vi "Main.vi"() -> ()   [LabVIEW 2020, in "Model.lvlib"]
doc: "This template is based off of the Queued Message Handler design pattern and the Queued Message Handler project template that ships with LabVIEW.\n\nThe main difference is that the queue is private to this module and communication between modules is performed via Broadcast and Request events.\n\nRequest events are wrapped in public API methods and are handled in the Event Handling Loop (EHL) of this VI. Any module can register for Broadcast events sent by this module. The EHL generates messages based on user interface actions.\n\nThe Message Handling Loop (MHL) processes messages generated by the EHL, or by other messages. The messages are string values, so new messages can be added easily to the Message Cases case structure in the MHL. Each message cluster can also provide an optional value for Message Data, which is a variant that can be converted to whatever message-specific data is required.\n_____\nBased on Delacor QMH Project Template 4.2.1.64."
uses:
  Model.lvlib
  <vilib>/Delacor/Delacor QMH/Libraries/Module Admin_class/Delacor_lib_QMH_Module Admin.lvclass
  Module Data--cluster.ctl
  <vilib>/Delacor/Delacor QMH/Libraries/Message Queue_class/Delacor_lib_QMH_Message Queue.lvclass/Delacor_lib_QMH_Message Queue.ctl
  Stop Argument--cluster.ctl
  <vilib>/Delacor/Delacor QMH/Libraries/Module Admin_class/Delacor_lib_QMH_Module Admin.lvclass/Delacor_lib_QMH_Module Admin.ctl
  <vilib>/Delacor/Delacor QMH/Libraries/Message Queue_class/Delacor_lib_QMH_Enqueue Message (Single).vi
  <vilib>/Delacor/Delacor QMH/Libraries/Module Admin_class/Delacor_lib_QMH_Get External Launch.vi
  <vilib>/Utility/error.llb/Error Cluster From Error Code.vi
  <vilib>/ErrorRing/Error Ring.xnode
  <vilib>/Delacor/Delacor QMH/Libraries/Message Queue_class/Delacor_lib_QMH_Message Queue.lvclass
  Stock/Stock.lvlib
  Display/Display.lvlib
  Keypad/Keypad.lvlib
  Money/Money.lvlib
panel:
  in  "Power":bool
  in  "Simulate MHL Error":bool
  in  "Simulate EHL Error":bool
  in  "Module Admin":refnum<class "Delacor_lib_QMH_Module Admin.lvclass">
  out "Status":string
  out "error out":errorcluster
  # "https://www.youtube.com/tomslabviewadventure | DQMH Vending Machine"
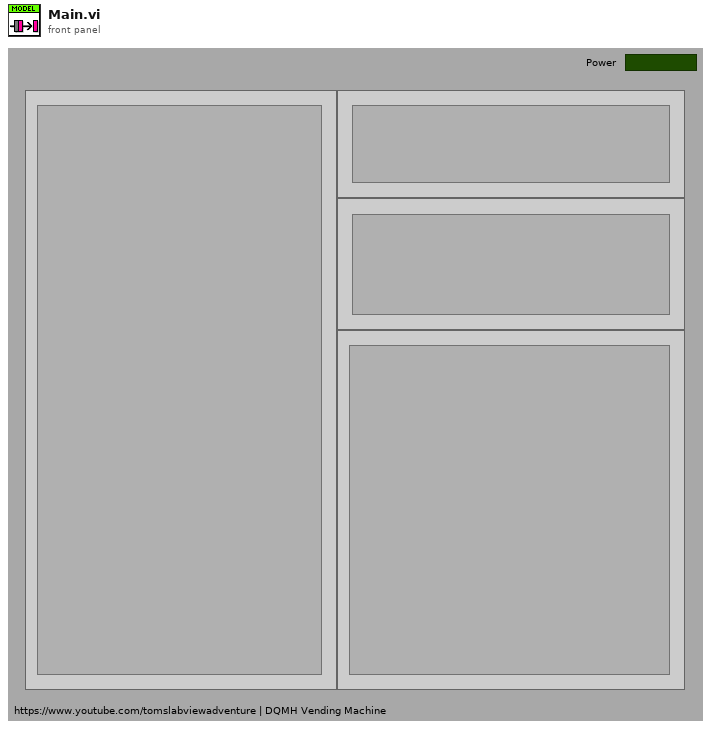
[diagram p1: front panel]
types:
  T1 = typedef "Model.lvlib/Request Events--cluster.ctl" = cluster{"Stop Module":refnum<user-event>, "Show Panel":refnum<user-event>, "Hide Panel":refnum<user-event>, "Get Module Execution Status":refnum<user-event>, "Show Diagram":refnum<user-event>}
  T2 = typedef "Stock.lvlib/Broadcast Events--cluster.ctl" = cluster{"Module Did Init":refnum<user-event>, "Status Updated":refnum<user-event>, "Error Reported":refnum<user-event>, "Module Did Stop":refnum<user-event>, "Update Module Execution Status":refnum<user-event>}
  T3 = typedef "Display.lvlib/Broadcast Events--cluster.ctl" = cluster{"Module Did Init":refnum<user-event>, "Status Updated":refnum<user-event>, "Error Reported":refnum<user-event>, "Module Did Stop":refnum<user-event>, "Update Module Execution Status":refnum<user-event>}
  T4 = typedef "Keypad.lvlib/Broadcast Events--cluster.ctl" = cluster{"Module Did Init":refnum<user-event>, "Status Updated":refnum<user-event>, "Error Reported":refnum<user-event>, "Module Did Stop":refnum<user-event>, "Update Module Execution Status":refnum<user-event>, "Product Selected":refnum<user-event>, "Cancel Request":refnum<user-event>}
  T5 = typedef "Money.lvlib/Broadcast Events--cluster.ctl" = cluster{"Module Did Init":refnum<user-event>, "Status Updated":refnum<user-event>, "Error Reported":refnum<user-event>, "Module Did Stop":refnum<user-event>, "Update Module Execution Status":refnum<user-event>, "Money Entered":refnum<user-event>, "Money Refunded":refnum<user-event>}
  T6 = typedef "Model.lvlib/Module Data--cluster.ctl" = cluster{"Status":string}
  T7 = enum32{"invalid lock state", "Not Locked", "Locked (No Password)", "Password-protected"}
  T8 = typedef "Model.lvlib/Stop Argument--cluster.ctl" = cluster{"Origin":string, "Exit via Stop Module Req?":bool, "Wait for Module to stop?":bool}
  T9 = enum32{"Invalid", "Standard", "Closed", "Hidden", "Minimized", "Maximized"}
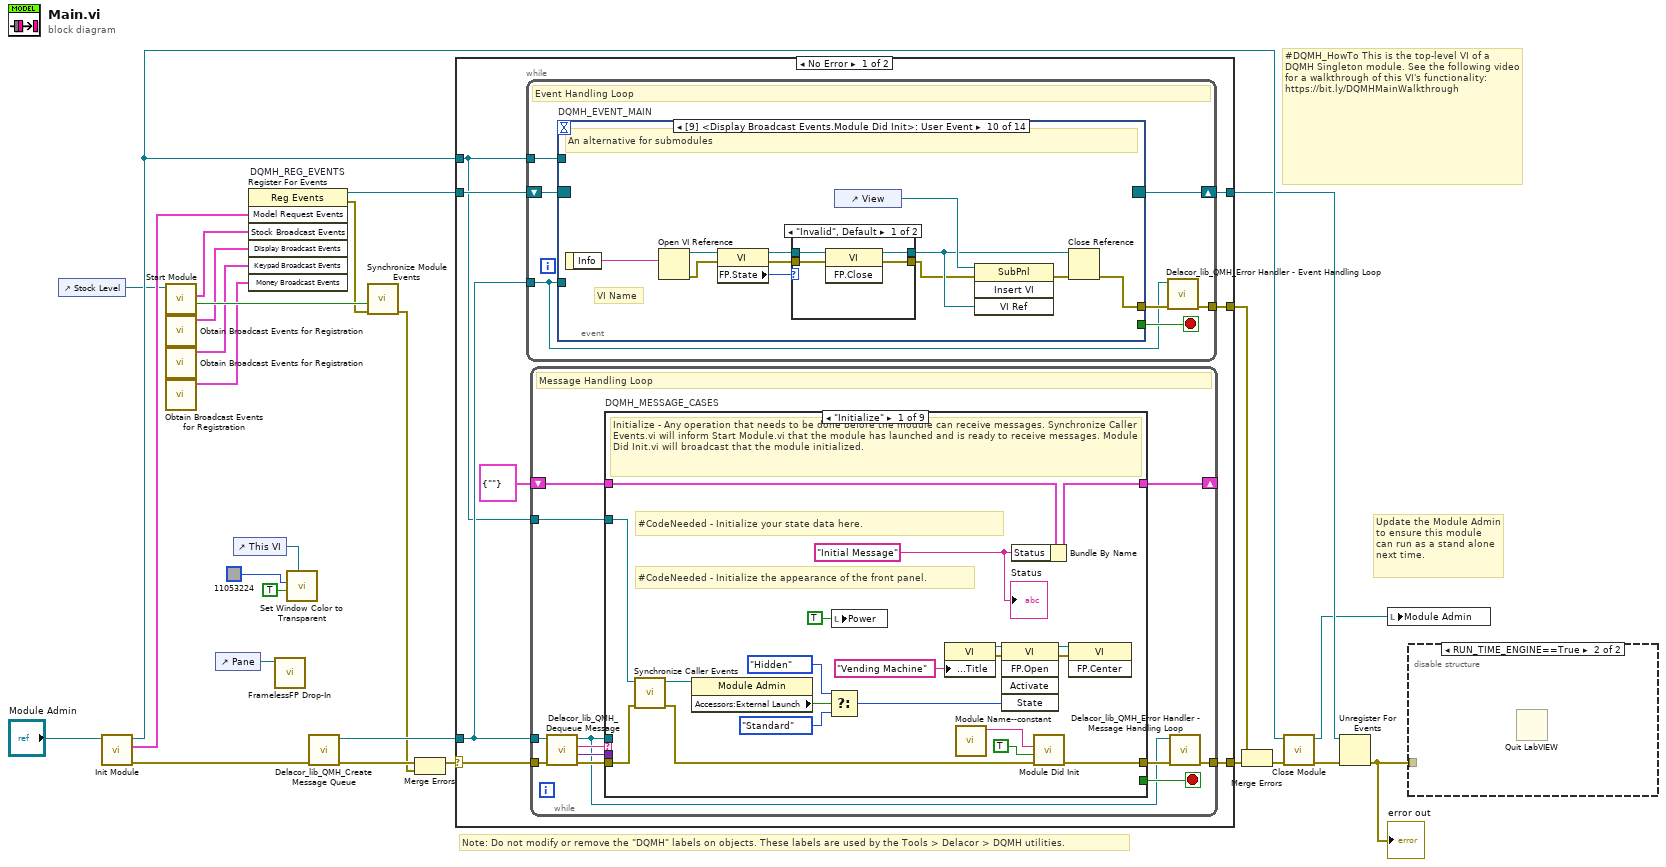
[diagram p0: block diagram]
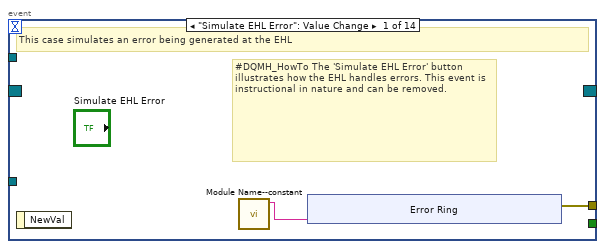
[diagram p3: hidden frame]
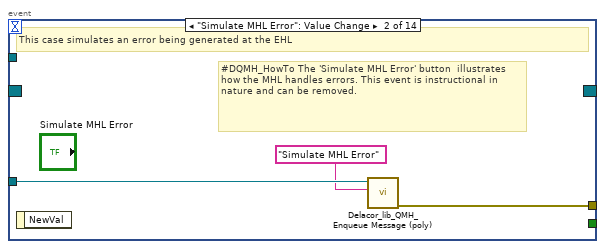
[diagram p4: hidden frame]
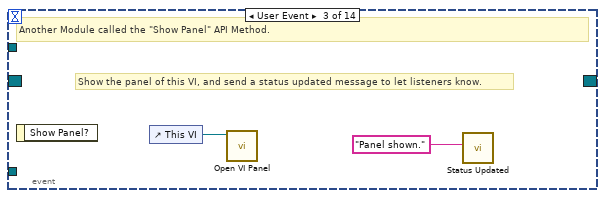
[diagram p5: hidden frame]
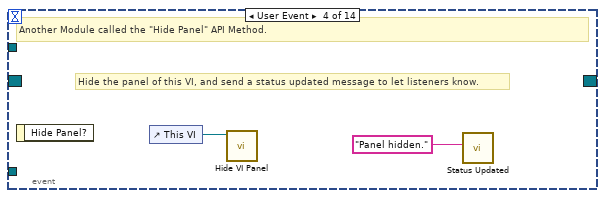
[diagram p6: hidden frame]
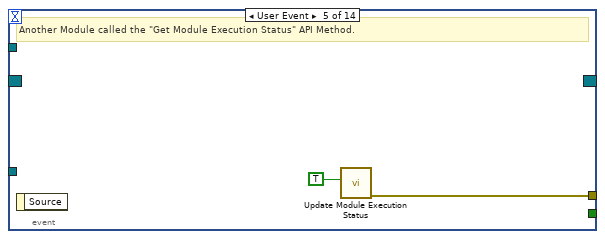
[diagram p7: hidden frame]
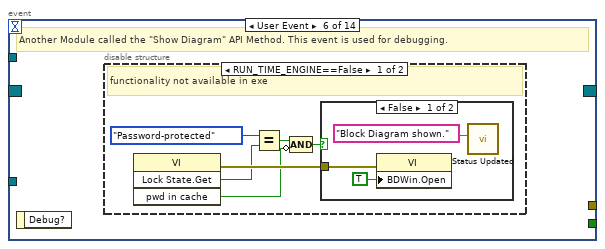
[diagram p8: hidden frame]
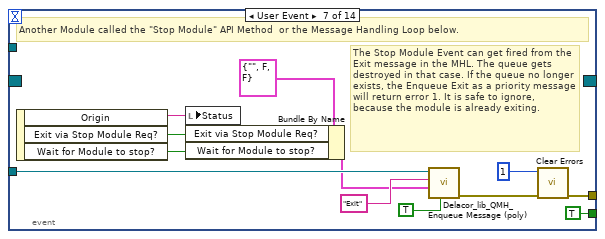
[diagram p11: hidden frame]
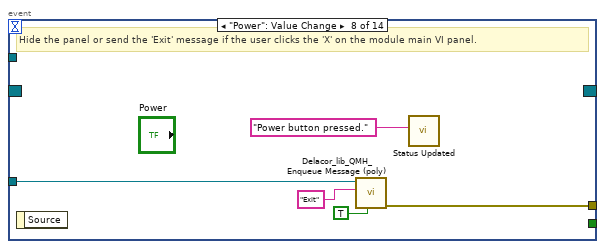
[diagram p12: hidden frame]
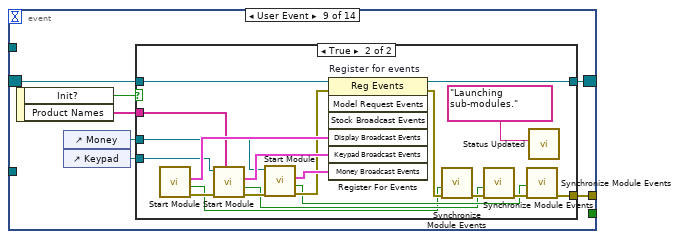
[diagram p13: hidden frame]
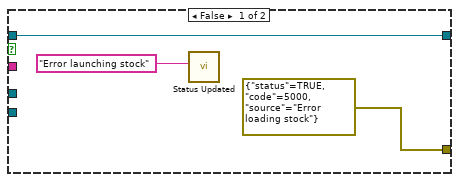
[diagram p14: hidden frame]
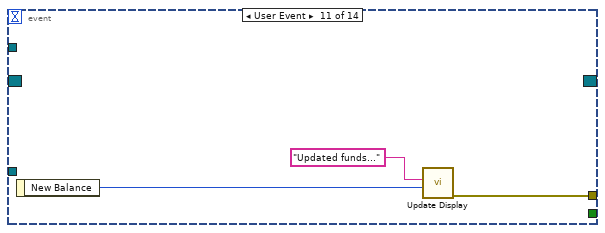
[diagram p16: hidden frame]
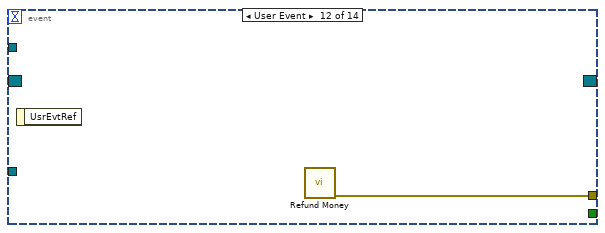
[diagram p17: hidden frame]
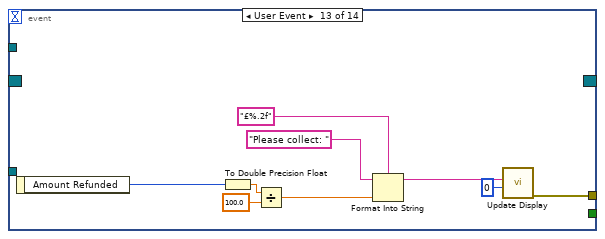
[diagram p18: hidden frame]
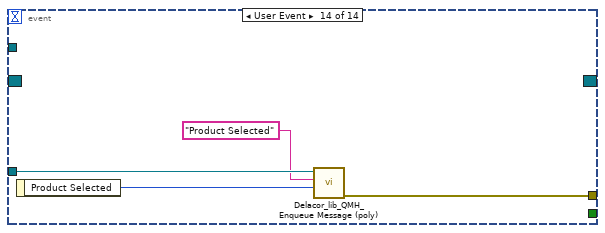
[diagram p19: hidden frame]
diagram:
  # "#DQMH_HowTo This is the top-level VI of a DQMH Singleton module. See the following video for a walkthrough of this VI's functionality: https://bit.ly/DQMHMainWalkthrough"
  # "Note: Do not modify or remove the \"DQMH\" labels on objects. These labels are used by the Tools > Delacor > DQMH utilities."
  # "Update the Module Admin to ensure this module can run as a stand alone next time."
  n1 = control-ref of="Stock Level"() -> (w6:refnum<vi>)
  n2 = call "Init Module.vi"("Singleton Module Admin in"="Module Admin") -> ("error out"=w26:errorcluster, "Model Request Events"=w17:T1, "Singleton Module Admin out"=w20:refnum<class "Delacor_lib_QMH_Module Admin.lvclass">)  [unwired: 8 in]
  n3 = call "Start Module.vi"("Subpanel Ref"=w6) -> ("Wait for Event Sync?"=w12:bool, "Stock Broadcast Events"=w13:T2)  [unwired: 7 in, 2 out]
  n4 = call "Obtain Broadcast Events for Registration.vi"() -> ("Display Broadcast Events"=w9:T3)  [unwired: 9 in, 2 out]
  n5 = call "Obtain Broadcast Events for Registration.vi"() -> ("Keypad Broadcast Events"=w8:T4)  [unwired: 9 in, 2 out]
  n6 = call "Obtain Broadcast Events for Registration.vi"() -> ("Money Broadcast Events"=w7:T5)  [unwired: 9 in, 2 out]
  n7 = control-ref of="Pane"() -> (w4:refnum<vi>)
  n8 = control-ref of="This VI"() -> (w1:refnum<vi>)
  n9 = register-events "DQMH_REG_EVENTS"(w17, w13, w9, w8, w7) -> (reference out=w18:refnum<event-registration>, error out=w11:errorcluster)  [unwired: 2 in]
  n10 = call "FramelessFP Drop-In.vi"("Pane in"=w4) -> ()  [unwired: 10 in, 1 out]
  n11 = call "Set Window Color to Transparent.vi"("Calling VI's reference"=w1, "Activate"=TRUE, "Color to Replace"=u32 11053224) -> ()  [unwired: 5 in, 1 out]
  n12 = call <vilib>:"Delacor_lib_QMH_Create Message Queue.vi"("error in"=w26) -> ("error out"=w22:errorcluster, "Message Queue"=w16:refnum<class "Delacor_lib_QMH_Message Queue.lvclass">)  [unwired: 9 in]
  n13 = call "Synchronize Module Events.vi"("error in (no error)"=w11, "Wait for Event Sync?"=w12) -> ("error out"=w10:errorcluster)  [unwired: 9 in]
  n14 = Merge Errors(w22, w10) -> (w21:errorcluster)
  n15 = case shown="No Error" w21 {
    selector: w21 -> [w33 w256]
    tunnel: [w35 w256] -> w27
    tunnel: [w32 w253] -> w19
    tunnel: w18 -> [w30 w253]
    tunnel: w16 -> [w29 _]
    tunnel: [w34 _] -> w24
    tunnel: w20 -> [w28 w249]
    frame No Error {
      n16 = while {
        tunnel: w29 -> [w36]
        shift-right: [w39] -> w32
        shift-left: w30 -> [w40]
        tunnel: [w41] -> w34
        tunnel: w28 -> [w37]
        stop <- w38 stop-if-true
        # "Event Handling Loop"
        n17 = event "DQMH_EVENT_MAIN" shown="[9] <Display Broadcast Events.Module Did Init>: User Event" {
          selector: w40 -> [_ _ _ _ _ _ _ _ w90 _ _ _ _ _]
          dyn-events: [_ _ _ _ _ _ _ _ w89 _ _ _ _ _] -> w39
          timeout: _ -> [_ _ _ _ _ _ _ _ _ _ _ _ _ _]
          tunnel: [_ _ _ _ _ _ TRUE ("Discard?") _ _ _ _ _ _ _] -> w38
          tunnel: w36 -> [_ w53 _ _ _ _ w77 w85 _ _ _ _ _ w149]
          tunnel: [w44 w54 _ _ w60 _ w80 w86 w92 w123 w135 w136 w145 w148] -> w42
          tunnel: w37 -> [_ _ _ _ _ _ _ _ _ _ _ _ _ _]
          event "Simulate EHL Error": Value Change {
            # "#DQMH_HowTo The 'Simulate EHL Error' button  illustrates how the EHL handles errors. This event is instructional in nature and can be removed."
            # "This case simulates an error being generated at the EHL"
            n18 = event-data() -> ()  [unwired: 1 in, 1 out]
            n19 = call "Module Name--constant.vi"() -> ("Module Name"=w43:string)  [unwired: 11 in]
            n20 = xnode "Error Ring"("parameter 0"=w43) -> ("error out"=w44:errorcluster)
          }
          event "Simulate MHL Error": Value Change {
            # "#DQMH_HowTo The 'Simulate MHL Error' button  illustrates how the MHL handles errors. This event is instructional in nature and can be removed."
            # "This case simulates an error being generated at the EHL"
            n21 = event-data() -> ()  [unwired: 1 in, 1 out]
            n22 = call-poly <vilib>:"Delacor_lib_QMH_Enqueue Message (poly).vi"("Message"="Simulate MHL Error", "Message Queue in"=w53) -> ("error out"=w54:errorcluster)  [unwired: 8 in, 1 out]
          }
          event User Event {
            # "Show the panel of this VI, and send a status updated message to let listeners know."
            # "Another Module called the \"Show Panel\" API Method."
            n23 = event-data() -> ()  [unwired: 1 in, 1 out]
            n24 = control-ref of="This VI"() -> (w56:refnum<vi>)
            n25 = call "Open VI Panel.vi"("VI"=w56) -> ()  [unwired: 10 in, 1 out]
            n26 = call "Status Updated.vi"("Status"="Panel shown." ("format string")) -> ()  [unwired: 10 in, 1 out]
          }
          event User Event {
            # "Hide the panel of this VI, and send a status updated message to let listeners know."
            # "Another Module called the \"Hide Panel\" API Method."
            n27 = event-data() -> ()  [unwired: 1 in, 1 out]
            n28 = control-ref of="This VI"() -> (w58:refnum<vi>)
            n29 = call "Hide VI Panel.vi"("VI"=w58) -> ()  [unwired: 10 in, 1 out]
            n30 = call "Status Updated.vi"("Status"="Panel hidden." ("format string")) -> ()  [unwired: 10 in, 1 out]
          }
          event User Event {
            # "Another Module called the \"Get Module Execution Status\" API Method."
            n31 = event-data() -> ()  [unwired: 1 in, 1 out]
            n32 = call "Update Module Execution Status.vi"("Running?"=TRUE) -> ("error out"=w60:errorcluster)  [unwired: 10 in]
          }
          event User Event {
            # "Another Module called the \"Show Diagram\" API Method. This event is used for debugging."
            n33 = event-data() -> ()  [unwired: 1 in, 1 out]
            n34 = disable-structure shown="RUN_TIME_ENGINE==False" {
              frame condition #0 (active) {
                # "functionality not available in exe"
                n35 = invoke class="VI" method="Lock State.Get"() -> (error out=w66:errorcluster, "Get Lock State"=w65:T7, "pwd in cache"=w62:bool)  [unwired: 4 in, 1 out]
                n36 = Equal?(x=T7."Password-protected", y=w65) -> (x = y?=w63:bool)
                n37 = Compound Arithmetic op=AND(w63, invert w62) -> (w61:bool)
                n38 = case shown="False" w61 {
                  tunnel: w66 -> [w69 _]
                  frame False {
                    n39 = property class="VI"(error in=w69, "BDWin.Open"=TRUE ("Block Diagram Window:Open")) -> ()  [unwired: 1 in, 2 out]
                    n40 = call "Status Updated.vi"("Status"="Block Diagram shown." ("format string")) -> ()  [unwired: 10 in, 1 out]
                  }
                  frame True {
                    # "Password-protected VI, and the password is not in the cache. Do not show the diagram."
                  }
                }
              }
              frame condition #1 {
              }
            }
          }
          event User Event {
            # "The Stop Module Event can get fired from the Exit message in the MHL. The queue gets destroyed in that case. If the queue no longer exists, the Enqueue Exit as a priority message will return error 1. It is safe to ignore, because the module is already exiting."
            # "Another Module called the \"Stop Module\" API Method  or the Message Handling Loop below."
            n41 = event-data() -> ("Origin"=w76:string, "Exit via Stop Module Req?"=w72:bool, "Wait for Module to stop?"=w71:bool)  [unwired: 1 in]
            n42 = local write "Status"(w76) -> ()
            n43 = Bundle By Name(cluster=T8 {"Origin"="", "Exit via Stop Module Req?"=FALSE, "Wait for Module to stop?"=FALSE} ("Stop Argument"), "Exit via Stop Module Req?"=w72, "Wait for Module to stop?"=w71) -> (w70:T8)
            n44 = call-poly <vilib>:"Delacor_lib_QMH_Enqueue Message (poly).vi"("Priority Message? (F)"=TRUE, "Message Data"=w70, "Message"="Exit", "Message Queue in"=w77) -> ("error out"=w81:errorcluster)  [unwired: 6 in, 1 out]
            n45 = call <vilib>:"Clear Errors.vi"("error in (no error)"=w81, "specific error code to clear (0: all)"=1) -> ("error out"=w80:errorcluster)  [unwired: 4 in, 1 out]
          }
          event "Power": Value Change {
            # "Hide the panel or send the 'Exit' message if the user clicks the 'X' on the module main VI panel."
            n46 = event-data() -> ()  [unwired: 1 in, 1 out]
            n47 = call-poly <vilib>:"Delacor_lib_QMH_Enqueue Message (poly).vi"("Priority Message? (F)"=TRUE, "Message"="Exit", "Message Queue in"=w85) -> ("error out"=w86:errorcluster)  [unwired: 7 in, 1 out]
            n48 = call "Status Updated.vi"("Status"="Power button pressed." ("format string")) -> ()  [unwired: 10 in, 1 out]
          }
          event User Event {
            n49 = event-data() -> ("Init?"=w93:bool, "Product Names"=w91:string[])  [unwired: 1 in]
            n50 = control-ref of="Money"() -> (w88:refnum<vi>)
            n51 = control-ref of="Keypad"() -> (w87:refnum<vi>)
            n52 = case shown="True" w93 {
              tunnel: [errorcluster {"status"=TRUE, "code"=5000, "source"="Error loading stock"} ("error constant") w104] -> w92
              tunnel: w91 -> [_ w100]
              tunnel: w90 -> [w95 w115]
              tunnel: [w95 w114] -> w89
              tunnel: w88 -> [_ w98]
              tunnel: w87 -> [_ w99]
              frame False {
                n53 = call "Status Updated.vi"("Status"="Error launching stock" ("format string")) -> ()  [unwired: 10 in, 1 out]
              }
              frame True {
                n54 = call "Start Module.vi"() -> ("error out"=w110:errorcluster, "Wait for Event Sync?"=w101:bool, "Display Broadcast Events"=w113:T3)  [unwired: 8 in, 1 out]
                n55 = call "Start Module.vi"("Product Names"=w100, "error in (no error)"=w110, "Subpanel Ref"=w99) -> ("error out"=w109:errorcluster, "Wait for Event Sync?"=w102:bool, "Keypad Broadcast Events"=w112:T4)  [unwired: 5 in, 1 out]
                n56 = call "Start Module.vi"("error in (no error)"=w109, "Subpanel Ref"=w98) -> ("error out"=w108:errorcluster, "Wait for Event Sync?"=w103:bool, "Money Broadcast Events"=w111:T5)  [unwired: 6 in, 1 out]
                n57 = register-events "Register for events"(reference=w115, error in=w108, w113, w112, w111) -> (reference out=w114:refnum<event-registration>, error out=w107:errorcluster)  [unwired: 2 in]
                n58 = call "Synchronize Module Events.vi"("error in (no error)"=w107, "Wait for Event Sync?"=w101) -> ("error out"=w106:errorcluster)  [unwired: 9 in]
                n59 = call "Synchronize Module Events.vi"("error in (no error)"=w106, "Wait for Event Sync?"=w102) -> ("error out"=w105:errorcluster)  [unwired: 9 in]
                n60 = call "Synchronize Module Events.vi"("error in (no error)"=w105, "Wait for Event Sync?"=w103) -> ("error out"=w104:errorcluster)  [unwired: 9 in]
                n61 = call "Status Updated.vi"("Status"="Launching sub-modules." ("format string")) -> ()  [unwired: 10 in, 1 out]
              }
            }
          }
          event User Event {
            # "VI Name"
            # "An alternative for submodules"
            n62 = event-data() -> ("Info"=w126:string)  [unwired: 1 in]
            n63 = Open VI Reference(vi path=w126) -> (vi reference=w122:refnum<vi>, error out=w119:errorcluster)  [unwired: 5 in]
            n64 = property class="VI"(reference=w122, error in=w119) -> (reference out=w120:refnum<vi>, error out=w118:errorcluster, "FP.State"=w121:T9)
            n65 = case shown="\"Invalid\", Default" w121 {
              tunnel: w120 -> [w130 w131]
              tunnel: w118 -> [w129 w132]
              tunnel: [w128 w132] -> w116
              tunnel: [w127 w131] -> w117
              frame "Invalid", Default {
                n66 = invoke class="VI" method="FP.Close"(reference=w130, error in=w129) -> (reference out=w127:refnum<vi>, error out=w128:errorcluster)  [unwired: 1 in, 1 out]
              }
              frame "Closed" {
              }
            }
            n67 = control-ref of="View"() -> (w125:refnum<vi>)
            n68 = invoke class="SubPnl" method="Insert VI"(reference=w125, error in=w116, "VI Ref"=w117) -> (error out=w124:errorcluster)  [unwired: 1 in, 3 out]
            n69 = Close Reference(reference=w117, error in (no error)=w124) -> (error out=w123:errorcluster)
          }
          event User Event {
            n70 = event-data() -> ("New Balance"=w134:u32)  [unwired: 1 in]
            n71 = call "Update Display.vi"("Balance"=w134, "Message to display"="Updated funds...") -> ("error out"=w135:errorcluster)  [unwired: 9 in]
          }
          event User Event {
            n72 = event-data() -> ()  [unwired: 1 in, 1 out]
            n73 = call "Refund Money.vi"() -> ("error out"=w136:errorcluster)  [unwired: 11 in]
          }
          event User Event {
            n74 = event-data() -> ("Amount Refunded"=w139:u32)  [unwired: 1 in]
            n75 = To Double Precision Float(number=w139) -> (double precision float=w142:dbl)
            n76 = Divide(x=w142, y=100.0) -> (x/y=w140:dbl)
            n77 = Format Into String(format string="£%.2f", initial string="Please collect: ", w140) -> (resulting string=w138:string)  [unwired: 1 in, 1 out]
            n78 = call "Update Display.vi"("Balance"=u32 0, "Message to display"=w138) -> ("error out"=w145:errorcluster)  [unwired: 9 in]
          }
          event User Event {
            n79 = event-data() -> ("Product Selected"=w146:u32)  [unwired: 1 in]
            n80 = call-poly <vilib>:"Delacor_lib_QMH_Enqueue Message (poly).vi"("Message Data"=w146, "Message"="Product Selected", "Message Queue in"=w149) -> ("error out"=w148:errorcluster)  [unwired: 7 in, 1 out]
          }
        }
        n81 = call-dynamic "Delacor_lib_QMH_Error Handler - Event Handling Loop.vi"("error in"=w42, "Message Queue in"=w36) -> ("dup error in"=w41:errorcluster)  [unwired: 8 in, 1 out]
      }
      n82 = while {
        tunnel: w29 -> [w152]
        shift-right: [w156] -> _
        shift-left: T6 {"Status"=""} ("Data Cluster") -> [w157]
        tunnel: w33 -> [w160]
        tunnel: [w158] -> w35
        tunnel: w28 -> [w150]
        stop <- w155 stop-if-true
        # "Message Handling Loop"
        n83 = call-dynamic "Delacor_lib_QMH_Dequeue Message.vi"("error in"=w160, "Message Queue in"=w152) -> ("error out"=w159:errorcluster, "Message Data"=w153:variant, "Message"=w154:string, "Message Queue out"=w151:refnum<class "Delacor_lib_QMH_Message Queue.lvclass">)  [unwired: 6 in]
        n84 = case "DQMH_MESSAGE_CASES" shown="\"Initialize\"" w154 {
          selector: w154 -> [_ _ _ _ _ _ _ _ w236]
          tunnel: w151 -> [_ _ _ _ _ _ w211 w228 _]
          tunnel: w159 -> [w179 w183 w186 w191 w195 w200 w218 w234 w238]
          tunnel: [w177 w183 w185 w187 w195 w199 w214 w231 w239] -> w161
          tunnel: w157 -> [w169 w182 w184 w193 w194 w197 w213 w227 w237]
          tunnel: [w168 w182 w184 w193 w194 w197 w213 w227 w237] -> w156
          tunnel: [_ _ _ _ _ _ _ w226 _] -> w155
          tunnel: w153 -> [_ _ _ w192 _ _ w212 w225 _]
          tunnel: w150 -> [w170 _ _ _ _ _ w210 w220 _]
          frame "Initialize" {
            w164 = "Initial Message" ("Initial Message")
            # "#CodeNeeded - Initialize the appearance of the front panel."
            # "#CodeNeeded - Initialize your state data here."
            # "Initialize - Any operation that needs to be done before the module can receive messages. Synchronize Caller Events.vi will inform Start Module.vi that the module has launched and is ready to receive messages. Module Did Init.vi will broadcast that the module initialized."
            n85 = call "Synchronize Caller Events.vi"("error in (no error)"=w179, "Singleton Module Admin in"=w170) -> ("error out"=w178:errorcluster, "Singleton Module Admin out"=w165:refnum<class "Delacor_lib_QMH_Module Admin.lvclass">)  [unwired: 8 in]
            n86 = property class="Module Admin"(reference=w165) -> ("Accessors:External Launch"=w174:bool)  [unwired: 1 in, 2 out]
            n87 = Select(t=T9."Hidden" ("State"), s=w174, f=T9."Standard" ("State")) -> (s? t:f=w171:T9)
            n88 = local write "Power"(TRUE ("Power")) -> ()
            n89 = property class="VI"("Front Panel.Title"="Vending Machine" ("Front Panel Window:Title")) -> (reference out=w176:refnum<vi>, error out=w181:errorcluster)  [unwired: 2 in]
            n90 = call "Module Name--constant.vi"() -> ("Module Name"=w166:string)  [unwired: 11 in]
            n91 = invoke class="VI" method="FP.Open"(reference=w176, error in=w181, "State"=w171) -> (reference out=w175:refnum<vi>, error out=w180:errorcluster)  [unwired: 2 in, 3 out]
            n92 = Bundle By Name(cluster=w169, "Status"=w164) -> (w168:T6)
            n93 = call "Module Did Init.vi"("error in (no error)"=w178, "Initialized?"=TRUE, "Origin"=w166) -> ("error out"=w177:errorcluster)  [unwired: 8 in]
            n94 = invoke class="VI" method="FP.Center"(reference=w175, error in=w180) -> ()  [unwired: 1 in, 3 out]
            "Status" <- w164
          }
          frame "--- Module Specific ---" {
            # "Separator -- The following cases handle messages specific to this Module."
          }
          frame "---Copy This Frame---" {
            # "Duplicate this frame when creating new messages.  Change this comment in the duplicated frame to describe this message."
            n95 = Merge Errors(w186) -> (w185:errorcluster)
          }
          frame "Product Selected" {
            # "All in one VI to reduce the risk of race conditions"
            # "Check Stock Level, Check Balance\nOutputs: Not in stock,  Insufficient Funds, Accepted (Reduce Stock and Balance"
            n96 = Variant To Data(error in=w191, type=u32 0 ("Product Selected"), Variant=w192) -> (data=w189:u32, error out=w188:errorcluster)
            n97 = call "Despence Product.vi"("error in (no error)"=w188, "Stock Item"=w189) -> ("error out"=w187:errorcluster)  [unwired: 9 in]
          }
          frame "--- Exit and Error Handling---" {
            # "Separator - The following cases handle errors and exit messages."
          }
          frame "Simulate MHL Error" {
            # "#DQMH_HowTo The 'Simulate MHL Error' button  illustrates how the MHL handles errors. This event is instructional in nature and can be removed."
            # "Simulate an error occurring at the MHL"
            n98 = call "Module Name--constant.vi"() -> ("Module Name"=w196:string)  [unwired: 11 in]
            n99 = xnode "Error Ring"("parameter 0"=w196) -> ("error out"=w198:errorcluster)
            n100 = Merge Errors(w200, w198) -> (w199:errorcluster)
          }
          frame "Error" {
            # "If the module is running standalone, then pop up an error dialog and call the \"Exit\" message."
            # "#CodeRecommended - If you ever change the name of this \"Error\" message, you'll need to update the name in the Check Loop Error.vi as well."
            # "#CodeRecommended - If the module is running in standalone mode (External Launch = FALSE), this code will pop up an error dialog and call the 'Exit' message if an error occurs. Add more fine-grained error handling here."
            # "Error - Check the error message data and respond accordingly. This message is sent by the \"Error Handler\" VIs at the end of each loop in this application."
            n101 = property class="Module Admin" props=["Accessors:External Launch"](reference=w210) -> ()  [unwired: 1 in, 3 out]
            n102 = Variant To Data(error in=w218, type=errorcluster {"status"=FALSE, "code"=0, "source"=""} ("error constant"), Variant=w212) -> (data=w219:errorcluster, error out=w216:errorcluster)
            n103 = call "Error Reported.vi"("Error"=w219) -> ()  [unwired: 10 in, 1 out]
            n104 = call <vilib>:"Simple Error Handler.vi"("error in (no error)"=w219) -> ()  [unwired: 4 in, 5 out]
            n105 = call-poly <vilib>:"Delacor_lib_QMH_Enqueue Message (poly).vi"("Priority Message? (F)"=TRUE, "Message"="Exit", "Message Queue in"=w211) -> ("error out"=w215:errorcluster)  [unwired: 7 in, 1 out]
            n106 = Merge Errors(w216, w215) -> (w214:errorcluster)
            n107 = local write "error out"(w214) -> ()
          }
          frame "Exit" {
            w224 = 91  # 91: not all Exit messages will have an argument
            w226 = TRUE  # Stop the VI
            # "Release the message queue reference"
            # "Exit - Exit the application."
            n108 = Variant To Data(error in=w234, type=T8 {"Origin"="", "Exit via Stop Module Req?"=FALSE, "Wait for Module to stop?"=FALSE} ("Stop Argument"), Variant=w225) -> (data=w222:T8, error out=w230:errorcluster)
            n109 = call <vilib>:"Clear Errors.vi"("error in (no error)"=w230, "specific error code to clear (0: all)"=w224) -> ("error out"=w233:errorcluster)  [unwired: 4 in, 1 out]
            n110 = control-ref of="This VI"() -> (w221:refnum<vi>)
            n111 = call-dynamic "Delacor_lib_QMH_Release Message Queue.vi"("error in"=w233, "Message Queue"=w228) -> ("error out"=w232:errorcluster)  [unwired: 9 in]
            n112 = call "Handle Exit.vi"("Stop Argument"=w222, "Admin in"=w220, "VI reference"=w221) -> ("error out"=w229:errorcluster)  [unwired: 7 in, 1 out]
            n113 = Merge Errors(w232, w229) -> (w231:errorcluster)
            n114 = call "Stop Module.vi"() -> ()  [unwired: 11 in, 1 out]
            n115 = call "Stop Module.vi"() -> ()  [unwired: 11 in, 1 out]
            n116 = call "Stop Module.vi"() -> ()  [unwired: 11 in, 1 out]
            n117 = call "Stop Module.vi"() -> ()  [unwired: 11 in, 1 out]
          }
          frame Default {
            # "'Default' case only runs if there is a message that isn't defined in any of the other cases.  Output a programming error."
            n118 = call "Module Name--constant.vi"() -> ("Module Name"=w235:string)  [unwired: 11 in]
            n119 = xnode "Error Ring"("parameter 0"=w236, "parameter 1"=w235) -> ("error out"=w240:errorcluster)
            n120 = Merge Errors(w238, w240) -> (w239:errorcluster)
          }
        }
        n121 = call-dynamic "Delacor_lib_QMH_Error Handler - Message Handling Loop.vi"("error in"=w161, "Message Queue in"=w151) -> ("dup error in"=w158:errorcluster)  [unwired: 8 in, 1 out]
      }
    }
    frame Error {
      # "Synchronize Caller Events.vi will inform Start Module.vi that the module has launched and will let the code calling Start Module.vi register for broadcasts and would permit the caller receive the broadcast that an error occurred at launch time."
      n122 = call "Synchronize Caller Events.vi"("Singleton Module Admin in"=w249) -> ("error out"=w254:errorcluster)  [unwired: 9 in, 1 out]
      n123 = call "Module Name--constant.vi"() -> ("Module Name"=w252:string)  [unwired: 11 in]
      n124 = Format Into String(format string="An error occurred during initialization. %s is no longer running.", w252) -> (resulting string=w250:string)  [unwired: 2 in, 1 out]
      n125 = Merge Errors(w256, w254) -> (w255:errorcluster)
      n126 = call "Error Reported.vi"("Additional Information"=w250, "Error"=w255) -> ()  [unwired: 9 in, 1 out]
    }
  }
  n127 = Merge Errors(w24, w27) -> (w23:errorcluster)
  n128 = call "Close Module.vi"("error in (no error)"=w23, "Module Admin in"=w20) -> ("error out"=w25:errorcluster, "Module Admin out"=w14:refnum<class "Delacor_lib_QMH_Module Admin.lvclass">)  [unwired: 7 in, 1 out]
  n129 = Unregister For Events(event registration refnum=w19, error in=w25) -> (error out=w5:errorcluster)
  "error out" <- w5
  n130 = local write "Module Admin"(w14) -> ()
  n131 = disable-structure shown="RUN_TIME_ENGINE==True" {
    disable-tunnel: w5 -> [_ _]
    frame condition #0 (active) {
    }
    frame condition #1 {
      n132 = Quit LabVIEW() -> ()  [unwired: 1 in]
    }
  }
